vi "cc_source.vi"(7 "Close":bool, 8 "error in (no error)":errorcluster, 11 "VISA":refnum<visa-resource-name>="tcpip0::192.168.1.5::5000::SOCKET") -> (0 "Error Out":errorcluster, 1 "Diode 3":dbl format="%.3f", 2 "Diode 2":dbl format="%.3f", 3 "Diode 1":dbl format="%.3f", 4 "Diode 4":dbl format="%.3f")   [LabVIEW 2020]
doc: "Cryocon Data Acquisition Example"
panel:
  in  "Serial Configuration":cluster{"Baud Rate":u32}={"Baud Rate"=9600} {"Baud Rate" items=["300"=300, "600"=600, "1200"=1200, "2400"=2400, "4800"=4800, "9600"=9600, "19200"=19200]}
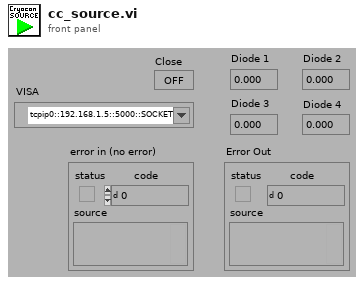
[diagram p1: front panel]
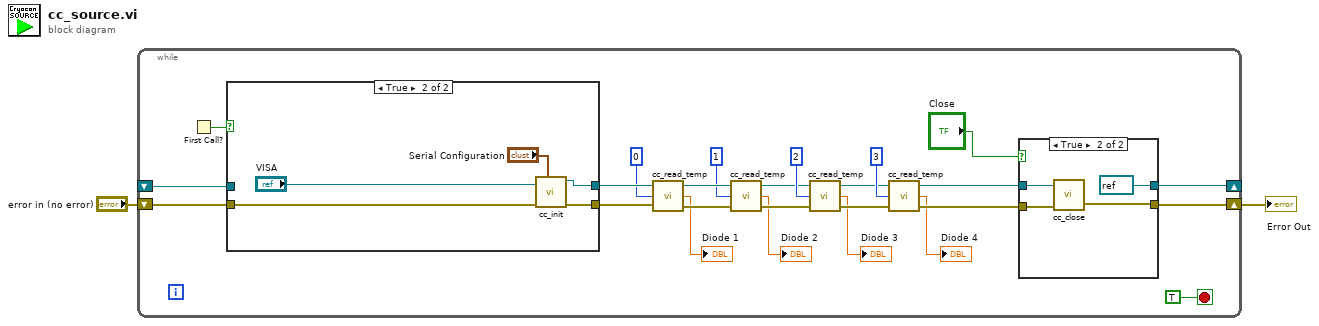
[diagram p0: block diagram]
diagram:
  n1 = while {
    shift-right: [w17] -> _
    shift-left: _ -> [w22]
    shift-right: [w18] -> w2
    shift-left: "error in (no error)" -> [w23]
    stop <- TRUE stop-if-true
    n2 = First Call?() -> (First Call?: T/F=w26:bool)
    n3 = case shown="True" w26 {
      tunnel: [w34 w39] -> w25
      tunnel: [w35 w38] -> w24
      tunnel: w23 -> [w35 w37]
      tunnel: w22 -> [w34 _]
      frame False {
      }
      frame True {
        n4 = call "cc_init.vi"("Serial Configuration"="Serial Configuration", "error in (no error)"=w37, "VISA resource name"="VISA") -> ("error out"=w38:errorcluster, "VISA resource name out"=w39:refnum<visa-resource-name>)  [unwired: 7 in]
      }
    }
    n5 = call "cc_read_temp.vi"("error in (no error)"=w24, "Input"=u8 0 ("Set Input 2"), "VISA In"=w25) -> ("error out"=w15:errorcluster, "Temperature"=→"Diode 1":dbl, "VISA Out"=w16:refnum<visa-resource-name>)
    n6 = call "cc_read_temp.vi"("error in (no error)"=w15, "Input"=u8 1 ("Set Input 2"), "VISA In"=w16) -> ("error out"=w7:errorcluster, "Temperature"=→"Diode 2":dbl, "VISA Out"=w8:refnum<visa-resource-name>)
    n7 = call "cc_read_temp.vi"("error in (no error)"=w7, "Input"=u8 2 ("Set Input 2"), "VISA In"=w8) -> ("error out"=w10:errorcluster, "Temperature"=→"Diode 3":dbl, "VISA Out"=w9:refnum<visa-resource-name>)
    n8 = call "cc_read_temp.vi"("error in (no error)"=w10, "Input"=u8 3 ("Set Input 2"), "VISA In"=w9) -> ("error out"=w19:errorcluster, "Temperature"=→"Diode 4":dbl, "VISA Out"=w21:refnum<visa-resource-name>)
    n9 = case shown="True" "Close" {
      tunnel: w21 -> [w28 w33]
      tunnel: w19 -> [w29 w32]
      tunnel: [w29 w31] -> w18
      tunnel: [w28 refnum<visa-resource-name> refnum ("VISA out")] -> w17
      frame False {
      }
      frame True {
        n10 = call "cc_close.vi"("error in (no error)"=w32, "VISA In"=w33) -> ("error out"=w31:errorcluster)  [unwired: 1 in]
      }
    }
  }
  "Error Out" <- w2
